vi "Get Most Recent Frame (if active).vi"(8 "error in (no error)":errorcluster, 11 "Andor Camera in":refnum<class "Andor Camera.lvclass">) -> (0 "error out":errorcluster, 3 "Andor Camera out":refnum<class "Andor Camera.lvclass">)   [LabVIEW 2023, in "Andor Camera.lvlib" / "Andor Camera.lvclass"]
uses:
  Andor Camera.lvclass
  C:/FlashGordon/Development/Hardware/Camera/Camera.lvclass
  C:/Program Files/National Instruments/LabVIEW 2023/vi.lib/ActorFramework/Actor/Actor.lvclass
  Andor Camera.lvclass/Andor Camera.ctl
  <vilib>/ActorFramework/Actor/Actor.lvclass/Actor.ctl
  Application Messages/New Frame Notify Msg/New Frame Notify Msg.lvclass/New Frame Notify Msg.ctl
  <vilib>/ActorFramework/Message Enqueuer/Message Enqueuer.lvclass/Message Enqueuer.ctl
  <vilib>/ActorFramework/Message Enqueuer/Enqueue.vi
  Application Messages/New Frame Notify Msg/New Frame Notify Msg.lvclass
  C:/Program Files/National Instruments/LabVIEW 2023/vi.lib/ActorFramework/Message/Message.lvclass
  Resources/GLOBAL/GLOBAL Time-critical.vi
  <vilib>/ActorFramework/Message Priority Queue/Priority Enqueue.vi
  Camera/Camera.lvlib
  <vilib>/ActorFramework/Actor/Actor.lvclass
panel:
  out "index":i32
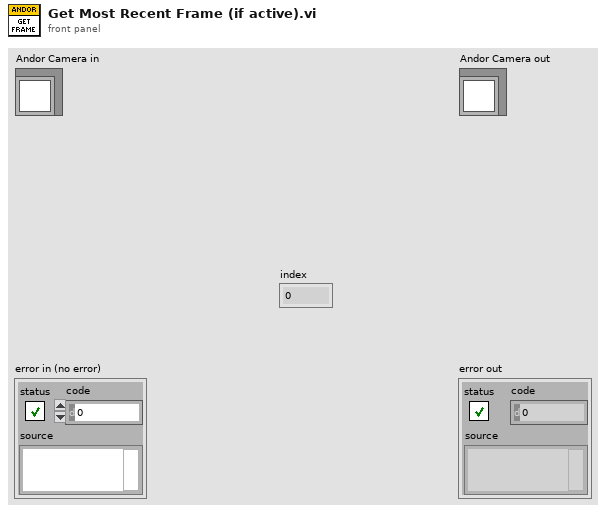
[diagram p1: front panel]
types:
  T1 = typedef "Physical Camera Assignment.ctl" = cluster{"Channel Name":string, "Serial Number":string, "Flip Vertically":bool, "Flip Horizontally":bool, "wavelength":i16, "photonsPerCount":dbl[]}
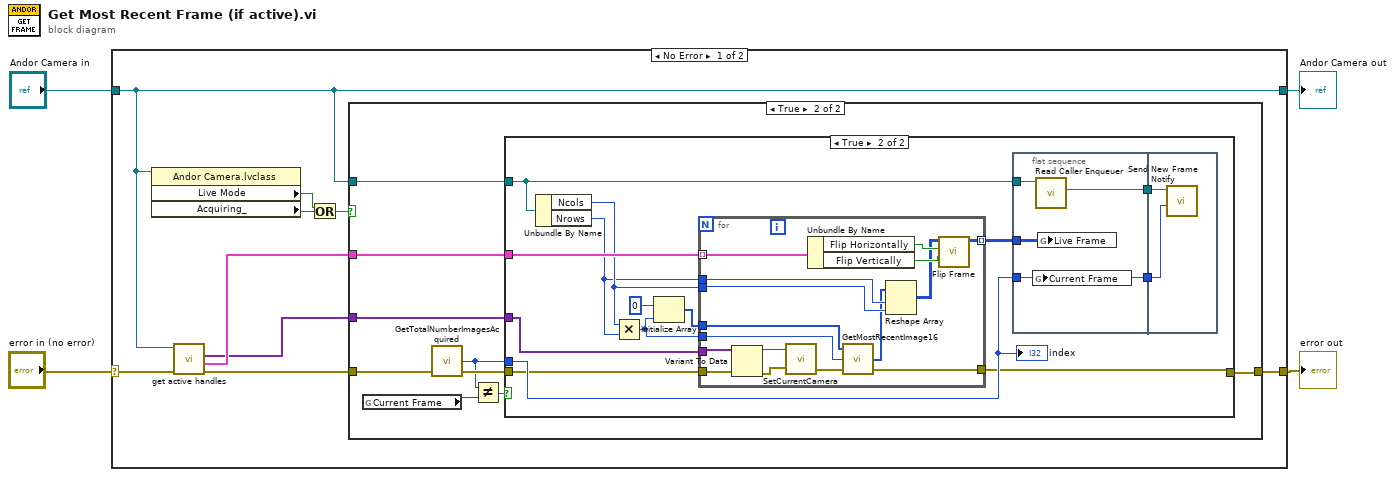
[diagram p0: block diagram]
diagram:
  n1 = case shown="No Error" "error in (no error)" {
    selector: "error in (no error)" -> [w10 w61]
    tunnel: [w11 w61] -> w2
    tunnel: "Andor Camera in" -> [w8 w62]
    tunnel: [w8 w62] -> w1
    frame No Error {
      n2 = property class="Andor Camera.lvclass"(reference=w8) -> ("Live Mode"=w13:bool, "Acquiring_"=w12:bool)  [unwired: 1 in, 2 out]
      n3 = call-dynamic "get active handles.vi"("error in (no error)"=w10, "Camera in"=w8) -> ("error out"=w5:errorcluster, "Active Cameras"=w9:T1[], "Handles"=w6:variant[])  [unwired: 5 in, 2 out]
      n4 = Or(x=w13, y=w12) -> (x .or. y?=w7:bool)
      n5 = case shown="True" w7 {
        tunnel: w5 -> [w14 w22]
        tunnel: [w14 w19] -> w11
        tunnel: w9 -> [_ w23]
        tunnel: w8 -> [_ w21]
        tunnel: w6 -> [_ w15]
        frame False {
        }
        frame True {
          n6 = global read "GLOBAL Time-critical.vi" "Current Frame"() -> (w18:i32)
          n7 = call <userlib>:"GetTotalNumberImagesAcquired.vi"("error in (no error)"=w22) -> ("error out"=w20:errorcluster, "index"=w17:i32)  [unwired: 2 in, 1 out]
          n8 = Not Equal?(x=w17, y=w18) -> (x != y?=w16:bool)
          n9 = case shown="True" w16 {
            tunnel: w23 -> [_ w36]
            tunnel: w21 -> [_ w34]
            tunnel: w20 -> [w24 w29]
            tunnel: [w24 w26] -> w19
            tunnel: w17 -> [_ w30]
            tunnel: w15 -> [_ w25]
            frame False {
            }
            frame True {
              n10 = Unbundle By Name(w34) -> ("Ncols"=w33:i32, "Nrows"=w32:i32)
              n11 = Multiply(x=w33, y=w32) -> (x*y=w28:i32)
              n12 = Initialize Array(u16 0, w28) -> (w27:u16[])
              n13 = for {
                tunnel: w36 -> [w60] mode=indexing
                tunnel: w33 -> [w54]
                tunnel: w32 -> [w56]
                tunnel: [w55] -> w35 mode=indexing
                tunnel: w29 -> [w48]
                tunnel: w28 -> [w53]
                tunnel: w27 -> [w52]
                tunnel: [w51] -> w26
                tunnel: w25 -> [w47]
                n14 = Variant To Data(error in=w48, Variant=w47) -> (data=w46:i32, error out=w45:errorcluster)  [unwired: 1 in]
                n15 = call <userlib>:"SetCurrentCamera.vi"("error in (no error)"=w45, "cameraHandle"=w46) -> ("error out"=w49:errorcluster)  [unwired: 1 out]
                n16 = Unbundle By Name(w60) -> ("Flip Horizontally"=w59:bool, "Flip Vertically"=w58:bool)
                n17 = call <userlib>:"GetMostRecentImage16.vi"("error in (no error)"=w49, "size"=w53, "array"=w52) -> ("error out"=w51:errorcluster, "array"=w50:u16[])  [unwired: 1 out]
                n18 = Reshape Array(w50, w56, w54) -> (w57:u16[][])
                n19 = call "Flip Frame.vi"("Flip Vertically"=w58, "Flip Horizontally"=w59, "Input Array"=w57) -> ("output array"=w55:u16[][])  [unwired: 8 in]
              }
              n20 = flat-sequence {
                tunnel: w35 -> [w42]
                tunnel: w34 -> [w41]
                tunnel: [w40] -> w38
                tunnel: w30 -> [w39]
                tunnel: [w39] -> w37
                tunnel: w38 -> [w44]
                tunnel: w37 -> [w43]
                frame #0 {
                  n21 = global write "GLOBAL Time-critical.vi" "Current Frame"(w39) -> ()
                  n22 = call <vilib>:"Read Caller Enqueuer.vi"("Actor"=w41) -> ("Caller Enqueuer"=w40:refnum<class "Message Enqueuer.lvclass">)  [unwired: 10 in]
                  n23 = global write "GLOBAL Time-critical.vi" "Live Frame"(w42) -> ()
                }
                frame #1 {
                  n24 = call "Send New Frame Notify.vi"("Frame Number\n(starts with 1)"=w43, "Message Enqueuer"=w44) -> ()  [unwired: 8 in, 2 out]
                }
              }
              "index" <- w30
            }
          }
        }
      }
    }
    frame Error {
    }
  }
  "error out" <- w2
  "Andor Camera out" <- w1
